vi "Cmd Get Parameter.vi"(4 "error in (no error)":errorcluster, 6 "parameter index":variant, 7 "command reference":T1) -> (0 "error out":errorcluster, 2 "ADODB.Parameter":refnum<k7>, 3 "command reference out":T1)   [LabVIEW 2013, in "NI_Database_API_64.lvlib"]
doc: "Returns a Parameter object refnum from the specified command reference."
uses:
  NI_Database_API_64.lvlib
  Cmd ObjectReference.ctl
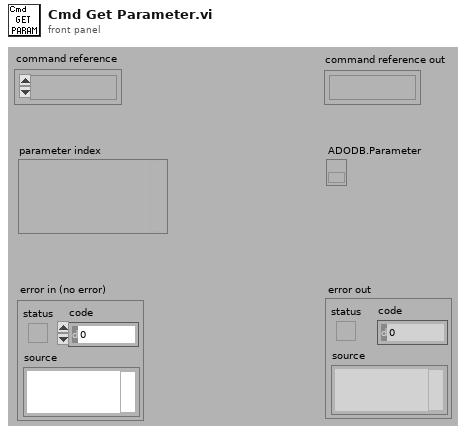
[diagram p1: front panel]
types:
  T1 = typedef "NI_Database_API_64.lvlib/Cmd ObjectReference.ctl" = refnum<k1>
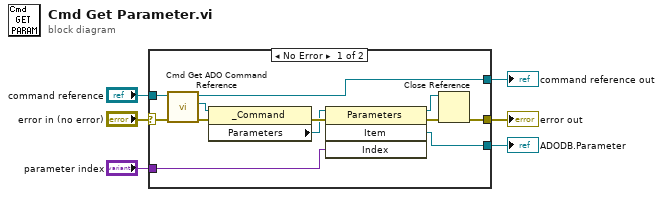
[diagram p0: block diagram]
diagram:
  n1 = case shown="No Error" "error in (no error)" {
    selector: "error in (no error)" -> [w7 w20]
    tunnel: "command reference" -> [w17 w19]
    tunnel: "parameter index" -> [w14 _]
    tunnel: [w13 w19] -> w4
    tunnel: [w10 w20] -> w3
    tunnel: [w9 _] -> w2
    frame No Error {
      n2 = call "Cmd Get ADO Command Reference.vi"("error in (no error)"=w7, "command reference"=w17) -> ("error out"=w15:errorcluster, "ADODB._Command"=w16:refnum<k7>, "command reference out"=w13:T1)  [unwired: 3 in]
      n3 = property class="_Command"(reference=w16, error in=w15) -> (error out=w18:errorcluster, "Parameters"=w8:refnum<k7>)  [unwired: 1 out]
      n4 = invoke class="Parameters" method="Item"(reference=w8, error in=w18, "Index"=w14) -> (reference out=w11:refnum<k7>, error out=w12:errorcluster, "Item"=w9:refnum<k7>)  [unwired: 1 in, 1 out]
      n5 = Close Reference(reference=w11, error in (no error)=w12) -> (error out=w10:errorcluster)
    }
    frame Error {
    }
  }
  "ADODB.Parameter" <- w2
  "error out" <- w3
  "command reference out" <- w4
